vi "Main.vi"(11 "Module Admin":refnum<class "Delacor_lib_QMH_Module Admin.lvclass">) -> ()   [LabVIEW 2020, in "UI.lvlib"]
doc: "This template is based off of the Queued Message Handler design pattern and the Queued Message Handler project template that ships with LabVIEW.\n\nThe main difference is that the queue is private to this module and communication between modules is performed via Broadcast and Request events.\n\nRequest events are wrapped in public API methods and are handled in the Event Handling Loop (EHL) of this VI. Any module can register for Broadcast events sent by this module. The EHL generates messages based on user interface actions.\n\nThe Message Handling Loop (MHL) processes messages generated by the EHL, or by other messages. The messages are string values, so new messages can be added easily to the Message Cases case structure in the MHL. Each message cluster can also provide an optional value for Message Data, which is a variant that can be converted to whatever message-specific data is required.\n_____\nBased on Delacor QMH Project Template 5.0.0.82."
uses:
  UI.lvlib
  <vilib>/Delacor/Delacor QMH/Libraries/Module Admin_class/Delacor_lib_QMH_Module Admin.lvclass
  Module Data--cluster.ctl
  Stop Argument--cluster.ctl
  <vilib>/Delacor/Delacor QMH/Libraries/Message Queue_class/Delacor_lib_QMH_Message Queue.lvclass/Delacor_lib_QMH_Message Queue.ctl
  <vilib>/Delacor/Delacor QMH/Libraries/Module Admin_class/Delacor_lib_QMH_Module Admin.lvclass/Delacor_lib_QMH_Module Admin.ctl
  <vilib>/Delacor/Delacor QMH/Libraries/Message Queue_class/Delacor_lib_QMH_Enqueue Message (Single).vi
  <vilib>/Delacor/Delacor QMH/Libraries/Module Admin_class/Delacor_lib_QMH_Get External Launch.vi
  <vilib>/Utility/error.llb/Error Cluster From Error Code.vi
  <vilib>/ErrorRing/Error Ring.xnode
  <vilib>/Delacor/Delacor QMH/Libraries/Message Queue_class/Delacor_lib_QMH_Message Queue.lvclass
  Productos/Productos.lvlib
  Messages/Messages.lvlib
  Coins/Coins.lvlib
  Config/Config.lvlib
panel:
  out "error out":errorcluster
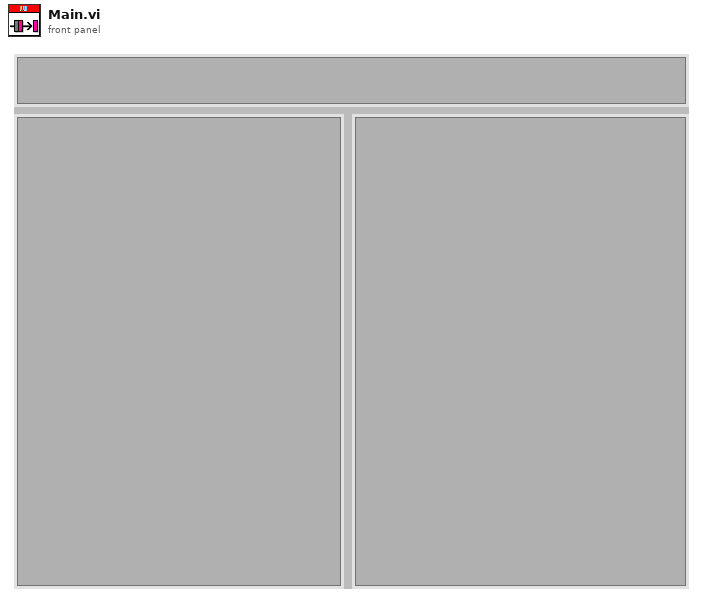
[diagram p1: front panel]
types:
  T1 = typedef "UI.lvlib/Request Events--cluster.ctl" = cluster{"Stop Module":refnum<user-event>, "Show Panel":refnum<user-event>, "Hide Panel":refnum<user-event>, "Get Module Execution Status":refnum<user-event>, "Show Diagram":refnum<user-event>}
  T2 = typedef "Config.lvlib/Broadcast Events--cluster.ctl" = cluster{"Module Did Init":refnum<user-event>, "Status Updated":refnum<user-event>, "Error Reported":refnum<user-event>, "Module Did Stop":refnum<user-event>, "Update Module Execution Status":refnum<user-event>}
  T3 = typedef "Productos.lvlib/Broadcast Events--cluster.ctl" = cluster{"Module Did Init":refnum<user-event>, "Status Updated":refnum<user-event>, "Error Reported":refnum<user-event>, "Module Did Stop":refnum<user-event>, "Update Module Execution Status":refnum<user-event>}
  T4 = typedef "Coins.lvlib/Broadcast Events--cluster.ctl" = cluster{"Module Did Init":refnum<user-event>, "Status Updated":refnum<user-event>, "Error Reported":refnum<user-event>, "Module Did Stop":refnum<user-event>, "Update Module Execution Status":refnum<user-event>}
  T5 = typedef "Messages.lvlib/Broadcast Events--cluster.ctl" = cluster{"Module Did Init":refnum<user-event>, "Status Updated":refnum<user-event>, "Error Reported":refnum<user-event>, "Module Did Stop":refnum<user-event>, "Update Module Execution Status":refnum<user-event>}
  T6 = typedef "UI.lvlib/Module Data--cluster.ctl" = cluster{"Status":string}
  T7 = enum32{"invalid lock state", "Not Locked", "Locked (No Password)", "Password-protected"}
  T8 = typedef "UI.lvlib/Stop Argument--cluster.ctl" = cluster{"Origin":string, "Exit via Stop Module Req?":bool, "Wait for Module to stop?":bool}
  T9 = enum32{"Invalid", "Standard", "Closed", "Hidden", "Minimized", "Maximized"}
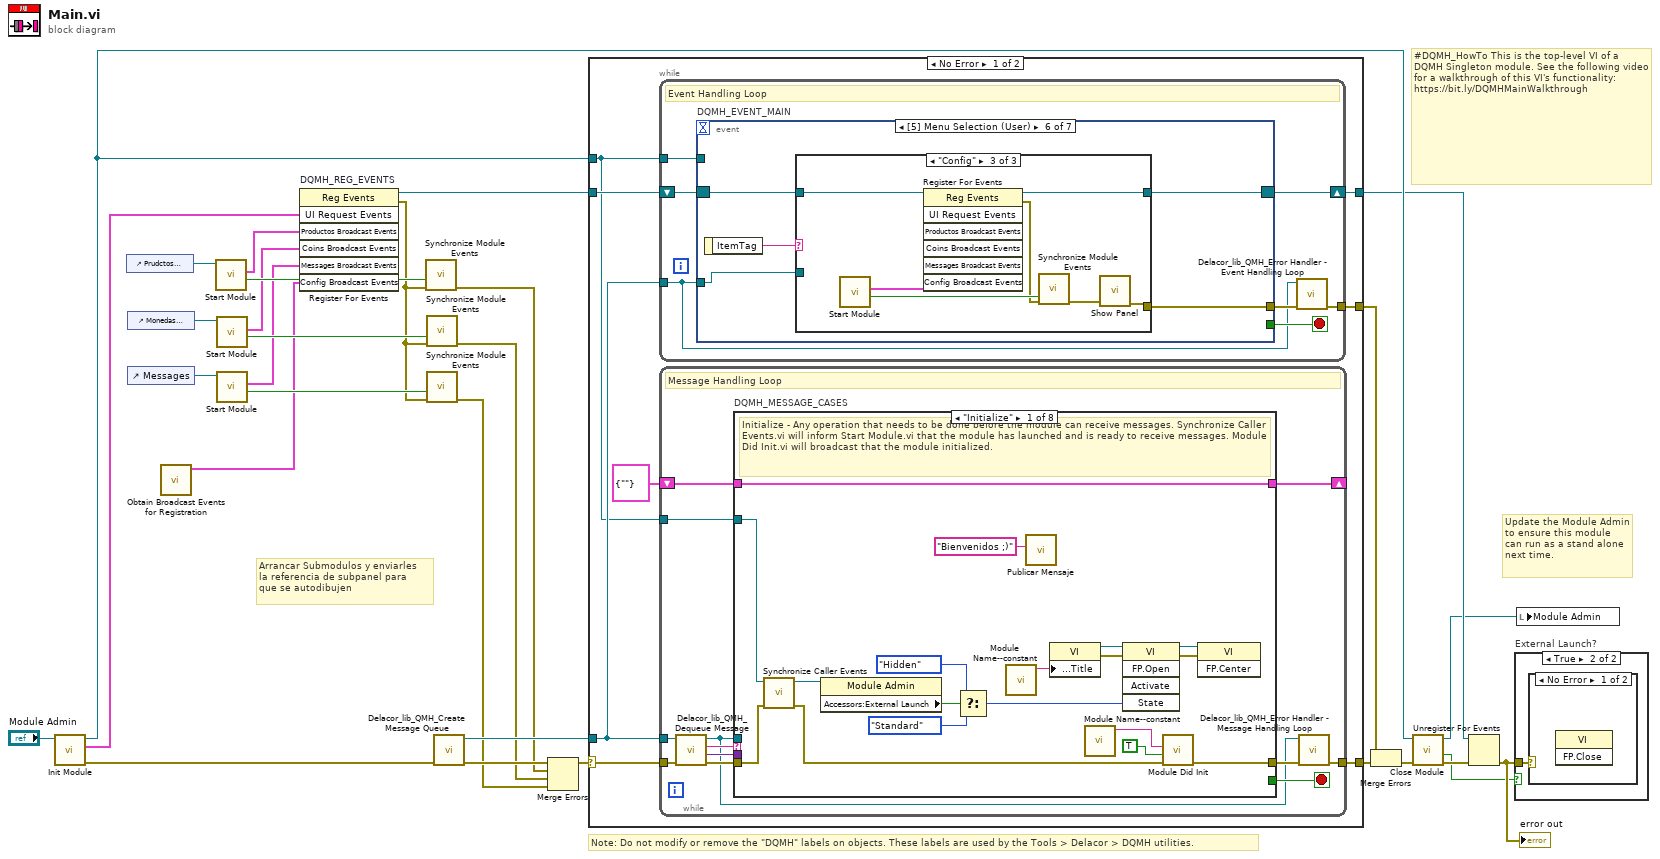
[diagram p0: block diagram]
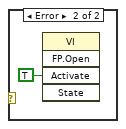
[diagram p3: hidden frame]
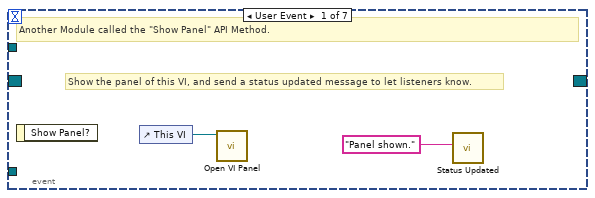
[diagram p4: hidden frame]
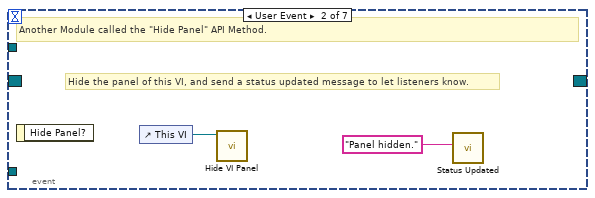
[diagram p5: hidden frame]
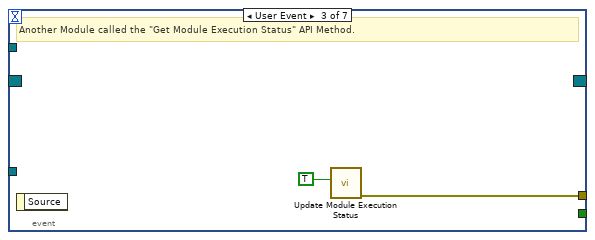
[diagram p6: hidden frame]
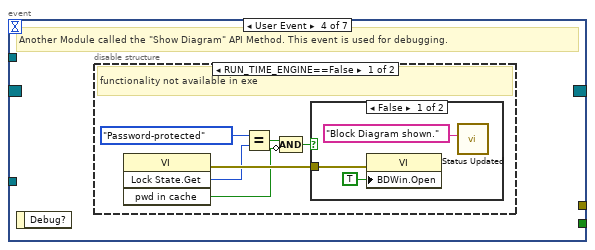
[diagram p7: hidden frame]
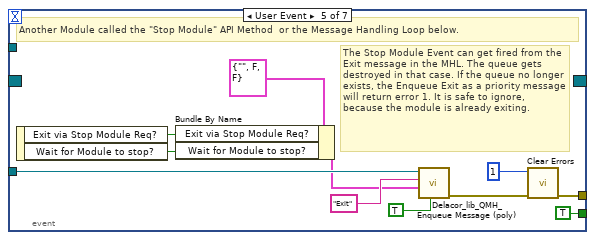
[diagram p10: hidden frame]
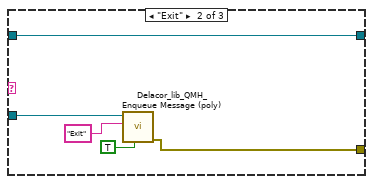
[diagram p12: hidden frame]
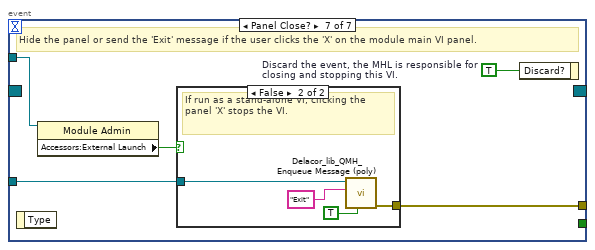
[diagram p13: hidden frame]
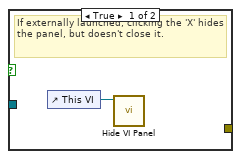
[diagram p14: hidden frame]
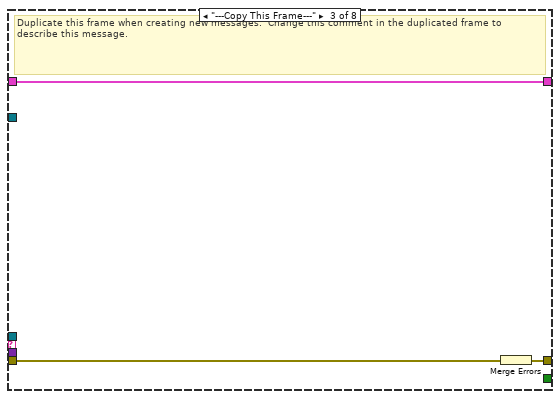
[diagram p16: hidden frame]
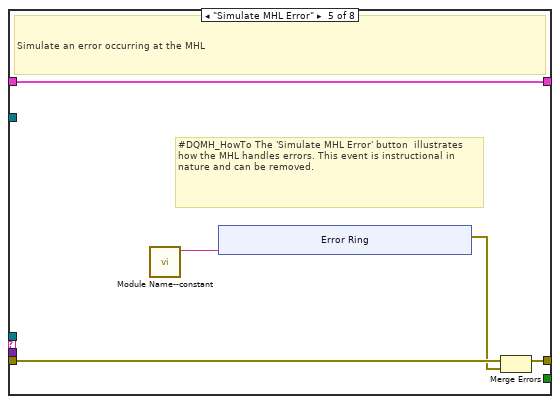
[diagram p18: hidden frame]
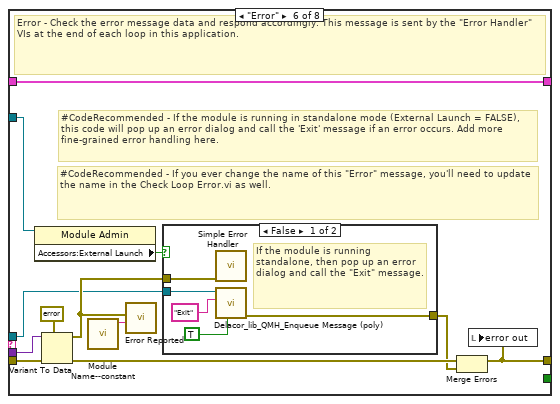
[diagram p19: hidden frame]
diagram:
  # "Arrancar Submodulos y enviarles\nla referencia de subpanel para\nque se autodibujen"
  # "#DQMH_HowTo This is the top-level VI of a DQMH Singleton module. See the following video for a walkthrough of this VI's functionality: https://bit.ly/DQMHMainWalkthrough"
  # "Note: Do not modify or remove the \"DQMH\" labels on objects. These labels are used by the Tools > Delacor > DQMH utilities."
  # "Update the Module Admin to ensure this module can run as a stand alone next time."
  n1 = call "Init Module.vi"("Singleton Module Admin in"="Module Admin") -> ("error out"=w29:errorcluster, "UI Request Events"=w19:T1, "Singleton Module Admin out"=w22:refnum<class "Delacor_lib_QMH_Module Admin.lvclass">)  [unwired: 8 in]
  n2 = control-ref of="Prudctos Subpanel"() -> (w11:refnum<vi>)
  n3 = control-ref of="Monedas Subpanel"() -> (w10:refnum<vi>)
  n4 = control-ref of="Messages"() -> (w9:refnum<vi>)
  n5 = call "Obtain Broadcast Events for Registration.vi"() -> ("Config Broadcast Events"=w1:T2)  [unwired: 9 in, 2 out]
  n6 = call "Start Module.vi"("Productos Subpanel"=w11) -> ("Wait for Event Sync?"=w14:bool, "Productos Broadcast Events"=w8:T3)  [unwired: 7 in, 2 out]
  n7 = call "Start Module.vi"("Monedas Subpanel"=w10) -> ("Wait for Event Sync?"=w13:bool, "Coins Broadcast Events"=w7:T4)  [unwired: 7 in, 2 out]
  n8 = call "Start Module.vi"("Messages Subpanel"=w9) -> ("Wait for Event Sync?"=w12:bool, "Messages Broadcast Events"=w6:T5)  [unwired: 7 in, 2 out]
  n9 = register-events "DQMH_REG_EVENTS"(w19, w8, w7, w6, w1) -> (reference out=w20:refnum<event-registration>, error out=w5:errorcluster)  [unwired: 2 in]
  n10 = call "Synchronize Module Events.vi"("error in (no error)"=w5, "Wait for Event Sync?"=w14) -> ("error out"=w4:errorcluster)  [unwired: 9 in]
  n11 = call "Synchronize Module Events.vi"("error in (no error)"=w5, "Wait for Event Sync?"=w13) -> ("error out"=w3:errorcluster)  [unwired: 9 in]
  n12 = call "Synchronize Module Events.vi"("error in (no error)"=w5, "Wait for Event Sync?"=w12) -> ("error out"=w2:errorcluster)  [unwired: 9 in]
  n13 = call <vilib>:"Delacor_lib_QMH_Create Message Queue.vi"("error in (no error)"=w29) -> ("error out"=w24:errorcluster, "Message Queue"=w18:refnum<class "Delacor_lib_QMH_Message Queue.lvclass">)  [unwired: 9 in]
  n14 = Merge Errors(w24, w4, w3, w2) -> (w23:errorcluster)
  n15 = case shown="No Error" w23 {
    selector: w23 -> [w36 w197]
    tunnel: [w38 w196] -> w30
    tunnel: [w35 w202] -> w21
    tunnel: w20 -> [w33 w202]
    tunnel: w18 -> [w32 w195]
    tunnel: [w37 _] -> w27
    tunnel: w22 -> [w31 w198]
    frame No Error {
      n16 = while {
        tunnel: w32 -> [w39]
        shift-right: [w42] -> w35
        shift-left: w33 -> [w43]
        tunnel: [w44] -> w37
        tunnel: w31 -> [w40]
        stop <- w41 stop-if-true
        # "Event Handling Loop"
        n17 = event "DQMH_EVENT_MAIN" shown="[5] Menu Selection (User)" {
          selector: w43 -> [_ _ _ _ _ w74 _]
          dyn-events: [_ _ _ _ _ w73 _] -> w42
          timeout: _ -> [_ _ _ _ _ _ _]
          tunnel: [_ _ _ _ TRUE ("Discard?") _ _] -> w41
          tunnel: w39 -> [_ _ _ _ w67 w75 w92]
          tunnel: [_ _ w51 _ w70 w72 w94] -> w45
          tunnel: w40 -> [_ _ _ _ _ _ w91]
          event User Event {
            # "Show the panel of this VI, and send a status updated message to let listeners know."
            # "Another Module called the \"Show Panel\" API Method."
            n18 = event-data() -> ()  [unwired: 1 in, 1 out]
            n19 = control-ref of="This VI"() -> (w47:refnum<vi>)
            n20 = call "Open VI Panel.vi"("VI"=w47) -> ()  [unwired: 10 in, 1 out]
            n21 = call "Status Updated.vi"("Status"="Panel shown." ("format string")) -> ()  [unwired: 10 in, 1 out]
          }
          event User Event {
            # "Hide the panel of this VI, and send a status updated message to let listeners know."
            # "Another Module called the \"Hide Panel\" API Method."
            n22 = event-data() -> ()  [unwired: 1 in, 1 out]
            n23 = control-ref of="This VI"() -> (w49:refnum<vi>)
            n24 = call "Hide VI Panel.vi"("VI"=w49) -> ()  [unwired: 10 in, 1 out]
            n25 = call "Status Updated.vi"("Status"="Panel hidden." ("format string")) -> ()  [unwired: 10 in, 1 out]
          }
          event User Event {
            # "Another Module called the \"Get Module Execution Status\" API Method."
            n26 = event-data() -> ()  [unwired: 1 in, 1 out]
            n27 = call "Update Module Execution Status.vi"("Running?"=TRUE) -> ("error out"=w51:errorcluster)  [unwired: 10 in]
          }
          event User Event {
            # "Another Module called the \"Show Diagram\" API Method. This event is used for debugging."
            n28 = event-data() -> ()  [unwired: 1 in, 1 out]
            n29 = disable-structure shown="RUN_TIME_ENGINE==False" {
              frame condition #0 (active) {
                # "functionality not available in exe"
                n30 = invoke class="VI" method="Lock State.Get"() -> (error out=w57:errorcluster, "Get Lock State"=w56:T7, "pwd in cache"=w53:bool)  [unwired: 4 in, 1 out]
                n31 = Equal?(x=T7."Password-protected", y=w56) -> (x = y?=w54:bool)
                n32 = Compound Arithmetic op=AND(w54, invert w53) -> (w52:bool)
                n33 = case shown="False" w52 {
                  tunnel: w57 -> [w60 _]
                  frame False {
                    n34 = property class="VI"(error in=w60, "BDWin.Open"=TRUE ("Block Diagram Window:Open")) -> ()  [unwired: 1 in, 2 out]
                    n35 = call "Status Updated.vi"("Status"="Block Diagram shown." ("format string")) -> ()  [unwired: 10 in, 1 out]
                  }
                  frame True {
                    # "Password-protected VI, and the password is not in the cache. Do not show the diagram."
                  }
                }
              }
              frame condition #1 {
              }
            }
          }
          event User Event {
            # "The Stop Module Event can get fired from the Exit message in the MHL. The queue gets destroyed in that case. If the queue no longer exists, the Enqueue Exit as a priority message will return error 1. It is safe to ignore, because the module is already exiting."
            # "Another Module called the \"Stop Module\" API Method  or the Message Handling Loop below."
            n36 = event-data() -> ("Exit via Stop Module Req?"=w63:bool, "Wait for Module to stop?"=w62:bool)  [unwired: 1 in]
            n37 = Bundle By Name(cluster=T8 {"Origin"="", "Exit via Stop Module Req?"=FALSE, "Wait for Module to stop?"=FALSE} ("Stop Argument"), "Exit via Stop Module Req?"=w63, "Wait for Module to stop?"=w62) -> (w61:T8)
            n38 = call-poly <vilib>:"Delacor_lib_QMH_Enqueue Message (poly).vi"("Priority Message? (F)"=TRUE, "Message Data"=w61, "Message"="Exit", "Message Queue in"=w67) -> ("error out"=w71:errorcluster)  [unwired: 6 in, 1 out]
            n39 = call <vilib>:"Clear Errors.vi"("error in (no error)"=w71, "specific error code to clear (0: all)"=1) -> ("error out"=w70:errorcluster)  [unwired: 4 in, 1 out]
          }
          event Menu Selection (User) {
            n40 = event-data() -> ("ItemTag"=w76:string)  [unwired: 1 in]
            n41 = case shown="\"Config\"" w76 {
              tunnel: w75 -> [_ w80 _]
              tunnel: w74 -> [w77 w79 w89]
              tunnel: [w77 w79 w87] -> w73
              tunnel: [_ w78 w83] -> w72
              frame "False", Default {
              }
              frame "Exit" {
                n42 = call-poly <vilib>:"Delacor_lib_QMH_Enqueue Message (poly).vi"("Priority Message? (F)"=TRUE, "Message"="Exit", "Message Queue in"=w80) -> ("error out"=w78:errorcluster)  [unwired: 7 in, 1 out]
              }
              frame "Config" {
                n43 = call "Start Module.vi"() -> ("Wait for Event Sync?"=w86:bool, "Config Broadcast Events"=w88:T2)  [unwired: 8 in, 2 out]
                n44 = register-events(reference=w89, w88) -> (reference out=w87:refnum<event-registration>, error out=w85:errorcluster)  [unwired: 5 in]
                n45 = call "Synchronize Module Events.vi"("error in (no error)"=w85, "Wait for Event Sync?"=w86) -> ("error out"=w84:errorcluster)  [unwired: 9 in]
                n46 = call "Show Panel.vi"("error in (no error)"=w84) -> ("error out"=w83:errorcluster)  [unwired: 10 in]
              }
            }
          }
          event Panel Close? {
            w93 = TRUE  # Discard the event, the MHL is responsible for closing and stopping this VI.
            # "Hide the panel or send the 'Exit' message if the user clicks the 'X' on the module main VI panel."
            n47 = event-data() -> ()  [unwired: 1 in, 1 out]
            n48 = property class="Module Admin"(reference=w91) -> ("Accessors:External Launch"=w90:bool)  [unwired: 1 in, 2 out]
            n49 = case shown="False" w90 {
              tunnel: w92 -> [_ w98]
              tunnel: [_ w99] -> w94
              frame True {
                # "If externally launched, clicking the 'X' hides the panel, but doesn't close it."
                n50 = control-ref of="This VI"() -> (w95:refnum<vi>)
                n51 = call "Hide VI Panel.vi"("VI"=w95) -> ()  [unwired: 10 in, 1 out]
              }
              frame False {
                # "If run as a stand-alone VI, clicking the panel 'X' stops the VI."
                n52 = call-poly <vilib>:"Delacor_lib_QMH_Enqueue Message (poly).vi"("Priority Message? (F)"=TRUE, "Message"="Exit", "Message Queue in"=w98) -> ("error out"=w99:errorcluster)  [unwired: 7 in, 1 out]
              }
            }
            n53 = event-data("Discard?"=w93) -> ()  [unwired: 1 in, 1 out]
          }
        }
        n54 = call-dynamic "Delacor_lib_QMH_Error Handler - Event Handling Loop.vi"("error in (no error)"=w45, "Message Queue in"=w39) -> ("dup error in"=w44:errorcluster)  [unwired: 8 in, 1 out]
      }
      n55 = while {
        tunnel: w32 -> [w102]
        shift-right: [w106] -> _
        shift-left: T6 {"Status"=""} ("Data Cluster") -> [w107]
        tunnel: w36 -> [w110]
        tunnel: [w108] -> w38
        tunnel: w31 -> [w100]
        stop <- w105 stop-if-true
        # "Message Handling Loop"
        n56 = call-dynamic "Delacor_lib_QMH_Dequeue Message.vi"("error in (no error)"=w110, "Message Queue in"=w102) -> ("error out"=w109:errorcluster, "Message Data"=w103:variant, "Message"=w104:string, "Message Queue out"=w101:refnum<class "Delacor_lib_QMH_Message Queue.lvclass">)  [unwired: 6 in]
        n57 = case "DQMH_MESSAGE_CASES" shown="\"Initialize\"" w104 {
          selector: w104 -> [_ _ _ _ _ _ _ w182]
          tunnel: w101 -> [_ _ _ _ _ w152 w174 _]
          tunnel: w109 -> [w127 w131 w134 w136 w141 w159 w180 w184]
          tunnel: [w125 w131 w133 w136 w140 w155 w177 w185] -> w111
          tunnel: w107 -> [w116 w130 w132 w135 w138 w154 w173 w183]
          tunnel: [w116 w130 w132 w135 w138 w154 w173 w183] -> w106
          tunnel: [_ _ _ _ _ _ w172 _] -> w105
          tunnel: w103 -> [_ _ _ _ _ w153 w171 _]
          tunnel: w100 -> [w117 _ _ _ _ w151 w166 _]
          frame "Initialize" {
            # "Initialize - Any operation that needs to be done before the module can receive messages. Synchronize Caller Events.vi will inform Start Module.vi that the module has launched and is ready to receive messages. Module Did Init.vi will broadcast that the module initialized."
            n58 = call "Synchronize Caller Events.vi"("error in (no error)"=w127, "Singleton Module Admin in"=w117) -> ("error out"=w126:errorcluster, "Singleton Module Admin out"=w113:refnum<class "Delacor_lib_QMH_Module Admin.lvclass">)  [unwired: 8 in]
            n59 = property class="Module Admin"(reference=w113) -> ("Accessors:External Launch"=w121:bool)  [unwired: 1 in, 2 out]
            n60 = Select(t=T9."Hidden" ("State"), s=w121, f=T9."Standard" ("State")) -> (s? t:f=w118:T9)
            n61 = call "Module Name--constant.vi"() -> ("Module Name"=w124:string)  [unwired: 11 in]
            n62 = call "Publicar Mensaje.vi"("Mensaje"="Bienvenidos ;)") -> ()  [unwired: 10 in, 1 out]
            n63 = property class="VI"("Front Panel.Title"=w124) -> (reference out=w123:refnum<vi>, error out=w129:errorcluster)  [unwired: 2 in]
            n64 = call "Module Name--constant.vi"() -> ("Module Name"=w114:string)  [unwired: 11 in]
            n65 = invoke class="VI" method="FP.Open"(reference=w123, error in=w129, "State"=w118) -> (reference out=w122:refnum<vi>, error out=w128:errorcluster)  [unwired: 2 in, 3 out]
            n66 = call "Module Did Init.vi"("error in (no error)"=w126, "Initialized?"=TRUE, "Origin"=w114) -> ("error out"=w125:errorcluster)  [unwired: 8 in]
            n67 = invoke class="VI" method="FP.Center"(reference=w122, error in=w128) -> ()  [unwired: 1 in, 3 out]
          }
          frame "--- Module Specific ---" {
            # "Separator -- The following cases handle messages specific to this Module."
          }
          frame "---Copy This Frame---" {
            # "Duplicate this frame when creating new messages.  Change this comment in the duplicated frame to describe this message."
            n68 = Merge Errors(w134) -> (w133:errorcluster)
          }
          frame "--- Exit and Error Handling---" {
            # "Separator - The following cases handle errors and exit messages."
          }
          frame "Simulate MHL Error" {
            # "#DQMH_HowTo The 'Simulate MHL Error' button  illustrates how the MHL handles errors. This event is instructional in nature and can be removed."
            # "Simulate an error occurring at the MHL"
            n69 = call "Module Name--constant.vi"() -> ("Module Name"=w137:string)  [unwired: 11 in]
            n70 = xnode "Error Ring"("parameter 0"=w137) -> ("error out"=w139:errorcluster)
            n71 = Merge Errors(w141, w139) -> (w140:errorcluster)
          }
          frame "Error" {
            # "#CodeRecommended - If you ever change the name of this \"Error\" message, you'll need to update the name in the Check Loop Error.vi as well."
            # "#CodeRecommended - If the module is running in standalone mode (External Launch = FALSE), this code will pop up an error dialog and call the 'Exit' message if an error occurs. Add more fine-grained error handling here."
            # "Error - Check the error message data and respond accordingly. This message is sent by the \"Error Handler\" VIs at the end of each loop in this application."
            n72 = property class="Module Admin"(reference=w151) -> ("Accessors:External Launch"=w150:bool)  [unwired: 1 in, 2 out]
            n73 = Variant To Data(error in=w159, type=errorcluster {"status"=FALSE, "code"=0, "source"=""} ("error constant"), Variant=w153) -> (data=w160:errorcluster, error out=w157:errorcluster)
            n74 = call "Module Name--constant.vi"() -> ("Module Name"=w149:string)  [unwired: 11 in]
            n75 = call "Error Reported.vi"("Additional Information"=w149, "Error"=w160) -> ()  [unwired: 9 in, 1 out]
            n76 = case shown="False" w150 {
              tunnel: [w165 _] -> w156
              tunnel: w152 -> [w163 _]
              tunnel: w160 -> [w164 _]
              frame False {
                # "If the module is running standalone, then pop up an error dialog and call the \"Exit\" message."
                n77 = call <vilib>:"Simple Error Handler.vi"("error in (no error)"=w164) -> ()  [unwired: 4 in, 5 out]
                n78 = call-poly <vilib>:"Delacor_lib_QMH_Enqueue Message (poly).vi"("Priority Message? (F)"=TRUE, "Message"="Exit", "Message Queue in"=w163) -> ("error out"=w165:errorcluster)  [unwired: 7 in, 1 out]
              }
              frame True {
                # "If the module was launched externally, calling the Error Reported broadcast VI is the only action performed by the \"Error\" message. The module's caller can then process the error appropriately."
              }
            }
            n79 = Merge Errors(w157, w156) -> (w155:errorcluster)
            n80 = local write "error out"(w155) -> ()
          }
          frame "Exit" {
            w170 = 91  # 91: not all Exit messages will have an argument
            w172 = TRUE  # Stop the VI
            # "Detener modulos"
            # "Release the message queue reference"
            # "#CodeNeeded - Add any required cleanup code here"
            # "Exit - Exit the application."
            n81 = Variant To Data(error in=w180, type=T8 {"Origin"="", "Exit via Stop Module Req?"=FALSE, "Wait for Module to stop?"=FALSE} ("Stop Argument"), Variant=w171) -> (data=w168:T8, error out=w176:errorcluster)
            n82 = call <vilib>:"Clear Errors.vi"("error in (no error)"=w176, "specific error code to clear (0: all)"=w170) -> ("error out"=w179:errorcluster)  [unwired: 4 in, 1 out]
            n83 = control-ref of="This VI"() -> (w167:refnum<vi>)
            n84 = call-dynamic "Delacor_lib_QMH_Release Message Queue.vi"("error in (no error)"=w179, "Message Queue"=w174) -> ("error out"=w178:errorcluster)  [unwired: 9 in]
            n85 = call "Handle Exit.vi"("Stop Argument"=w168, "Admin in"=w166, "VI reference"=w167) -> ("error out"=w175:errorcluster)  [unwired: 7 in, 1 out]
            n86 = Merge Errors(w178, w175) -> (w177:errorcluster)
            n87 = call "Stop Module.vi"() -> ()  [unwired: 11 in, 1 out]
            n88 = call "Stop Module.vi"() -> ()  [unwired: 11 in, 1 out]
            n89 = call "Stop Module.vi"() -> ()  [unwired: 11 in, 1 out]
          }
          frame Default {
            # "'Default' case only runs if there is a message that isn't defined in any of the other cases.  Output a programming error."
            n90 = call "Module Name--constant.vi"() -> ("Module Name"=w181:string)  [unwired: 11 in]
            n91 = xnode "Error Ring"("parameter 0"=w182, "parameter 1"=w181) -> ("error out"=w186:errorcluster)
            n92 = Merge Errors(w184, w186) -> (w185:errorcluster)
          }
        }
        n93 = call-dynamic "Delacor_lib_QMH_Error Handler - Message Handling Loop.vi"("error in (no error)"=w111, "Message Queue in"=w101) -> ("dup error in"=w108:errorcluster)  [unwired: 8 in, 1 out]
      }
    }
    frame Error {
      # "Synchronize Caller Events.vi will inform Start Module.vi that the module has launched and will let the code calling Start Module.vi register for broadcasts and would permit the caller receive the broadcast that an error occurred at launch time."
      n94 = call-dynamic "Delacor_lib_QMH_Release Message Queue.vi"("error in (no error)"=w197, "Message Queue"=w195) -> ("error out"=w196:errorcluster)  [unwired: 9 in]
      n95 = call "Synchronize Caller Events.vi"("Singleton Module Admin in"=w198) -> ("error out"=w203:errorcluster)  [unwired: 9 in, 1 out]
      n96 = call "Module Name--constant.vi"() -> ("Module Name"=w201:string)  [unwired: 11 in]
      n97 = Format Into String(format string="An error occurred during initialization. %s is no longer running.", w201) -> (resulting string=w199:string)  [unwired: 2 in, 1 out]
      n98 = Merge Errors(w196, w203) -> (w204:errorcluster)
      n99 = call "Error Reported.vi"("Additional Information"=w199, "Error"=w204) -> ()  [unwired: 9 in, 1 out]
    }
  }
  n100 = Merge Errors(w27, w30) -> (w26:errorcluster)
  n101 = call "Close Module.vi"("error in (no error)"=w26, "Module Admin in"=w22) -> ("error out"=w28:errorcluster, "External Launch"=w15:bool, "Module Admin out"=w16:refnum<class "Delacor_lib_QMH_Module Admin.lvclass">)  [unwired: 7 in]
  n102 = Unregister For Events(event registration refnum=w21, error in=w28) -> (error out=w25:errorcluster)
  "error out" <- w25
  n103 = case "External Launch?" shown="True" w15 {
    tunnel: w25 -> [_ w205]
    frame False {
    }
    frame True {
      n104 = case shown="No Error" w205 {
        frame No Error {
          n105 = invoke class="VI" method="FP.Close"() -> ()  [unwired: 3 in, 3 out]
        }
        frame Error {
          n106 = invoke class="VI" method="FP.Open"("Activate"=TRUE ("Activate?")) -> ()  [unwired: 4 in, 5 out]
        }
      }
    }
  }
  n107 = local write "Module Admin"(w16) -> ()
